vi "Simple Capture Move Stage.vi"(9 "Byte Stream File in":refnum<file>, 10 "Z Step Size (µm)":dbl, 11 "Notifier Name":string) -> ()   [LabVIEW 2016]
uses:
  Device Library/Stages/Stages Controls/Stage Actions.ctl
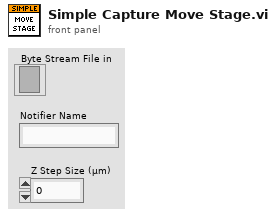
[diagram p1: front panel]
types:
  T1 = typedef "Stage Actions.ctl" = enum16{"Get Position", "MVR", "MOVE", "HALT", "ONTARGET", "ERROR", "REFERENCE", "INIT", "VELOCITY", "STATUS", "EXIT", "HOME", "ZEROPOS", "NANOPOS", "ANALOG", "QUIT"}
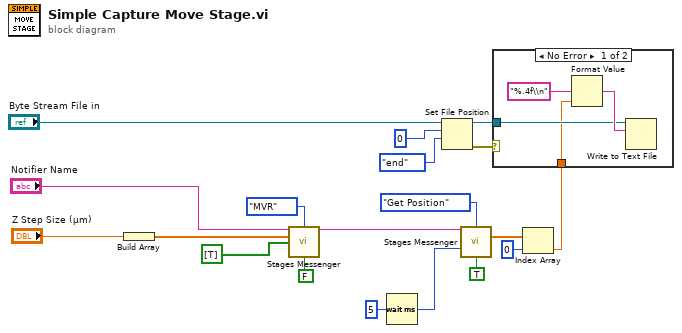
[diagram p0: block diagram]
diagram:
  n1 = Build Array("Z Step Size (µm)") -> (w4:dbl[])
  n2 = call "Stages Messenger.vi"("Stage Notifier Name"="Notifier Name", "Actions"=Stage_Actions."MVR", "Setpoint"=w4, "Axis"=bool[] [TRUE], "Exit While Busy?"=FALSE) -> ("Stage Notifier Name (Dup)"=w16:string)  [unwired: 7 in, 3 out]
  n3 = Wait (ms)(milliseconds to wait=u32 5) -> (millisecond timer value=w19:u32)
  n4 = Set File Position(offset (in bytes) (0)=i64 0, refnum="Byte Stream File in", from (0:start)=enum16{"start", "end", "current"}."end") -> (refnum out=w13:refnum<file>, error out=w15:errorcluster)  [unwired: 1 in]
  n5 = call "Stages Messenger.vi"("Stage Notifier Name"=w16, "Actions"=Stage_Actions."Get Position", "Velocity"=w19, "Exit While Busy?"=TRUE) -> ("Positions"=w9:dbl[])  [unwired: 8 in, 3 out]
  n6 = Index Array(array=w9, index=0) -> (element=w14:dbl)
  n7 = case shown="No Error" w15 {
    tunnel: w13 -> [w21 _]
    tunnel: w14 -> [w20 _]
    frame No Error {
      n8 = Format Value(format string="%.4f\\n", value (0)=w20) -> (output string=w23:string)  [unwired: 1 in]
      n9 = Write to Text File(file (use dialog)=w21, text=w23) -> ()  [unwired: 2 in, 3 out]
    }
    frame Error {
    }
  }
